vi "Basic serial write and or read.vi"(7 "ms to wait (150)":u32=150, 8 "error in (no error)":errorcluster, 9 "write string":string, 10 "action":T1(ring), 11 "VISA resource name":refnum<visa-resource-name>) -> (0 "error out":errorcluster, 1 "read string array":string[](array[string]), 2 "read string":string, 3 "VISA resource name out":refnum<visa-resource-name>)   [LabVIEW 2017, in "Millennia V.lvclass"]
doc: "Simplifies performing a basic read, write, or write + read to a device connected via serial port. It will read all messages waiting at the port and return them in an array. If you only expect a single message, use the \"read string\" output; otherwise, use the \"read string array\" output."
uses:
  Millennia V.lvclass
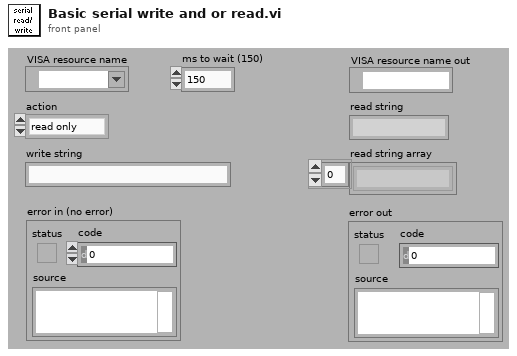
[diagram p1: front panel]
types:
  T1 = enum16{"read only", "write only", "write + read"}
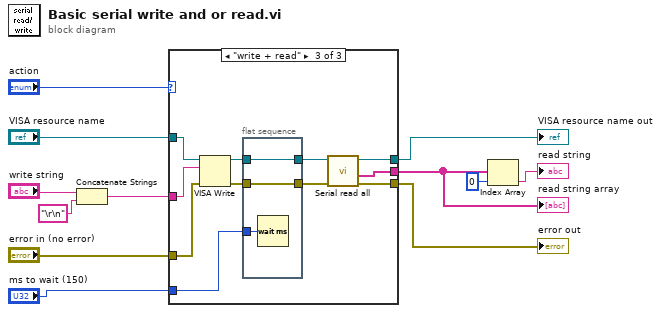
[diagram p0: block diagram]
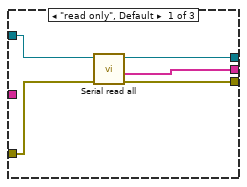
[diagram p2: hidden frame]
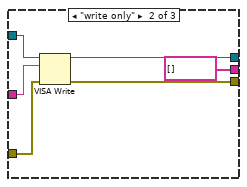
[diagram p3: hidden frame]
diagram:
  n1 = Concatenate Strings("write string", "\r\n" ("string")) -> (w8:string)
  n2 = case shown="\"write + read\"" "action" {
    tunnel: "error in (no error)" -> [w13 w21 w32]
    tunnel: w8 -> [_ w22 w33]
    tunnel: "VISA resource name" -> [w14 w23 w34]
    tunnel: [w17 w20 w25] -> w5
    tunnel: [w16 w19 w27] -> w4
    tunnel: [w15 string[] [] ("read string array 2") w24] -> w3
    tunnel: "ms to wait (150)" -> [_ _ w29]
    frame "read only", Default {
      n3 = call "Serial read all.vi"("error in (no error)"=w13, "VISA resource name"=w14) -> ("error out"=w16:errorcluster, "read strings"=w15:string[], "VISA resource name out"=w17:refnum<visa-resource-name>)  [unwired: 7 in]
    }
    frame "write only" {
      n4 = VISA Write(VISA resource name=w23, write buffer=w22, error in (no error)=w21) -> (VISA resource name out=w20:refnum<visa-resource-name>, error out=w19:errorcluster)  [unwired: 1 out]
    }
    frame "write + read" {
      n5 = VISA Write(VISA resource name=w34, write buffer=w33, error in (no error)=w32) -> (VISA resource name out=w30:refnum<visa-resource-name>, error out=w31:errorcluster)  [unwired: 1 out]
      n6 = flat-sequence {
        tunnel: w31 -> [w36]
        tunnel: w30 -> [w37]
        tunnel: [w37] -> w26
        tunnel: [w36] -> w28
        tunnel: w29 -> [w35]
        frame #0 {
          n7 = Wait (ms)(milliseconds to wait=w35) -> ()  [unwired: 1 out]
        }
      }
      n8 = call "Serial read all.vi"("error in (no error)"=w28, "VISA resource name"=w26) -> ("error out"=w27:errorcluster, "read strings"=w24:string[], "VISA resource name out"=w25:refnum<visa-resource-name>)  [unwired: 7 in]
    }
  }
  "VISA resource name out" <- w5
  "error out" <- w4
  "read string array" <- w3
  n9 = Index Array(array=w3, index=0) -> (element=→"read string":string)
